vi "nanocal -- nuclear schottky fit -- 2x2 -- V9.vi"() -> ()   [LabVIEW 2021] (continued)
\"τC\" -> 0.000000000000   ,  \"κ0\" -> 0.000000000000   ,  \"mm1\" -> 0.000000000000   ,  \"mm2\" -> 0.000000000000   ,  \"mm3\" -> 0.000000000000   ,  \"T\" -> 3.070000000000   ,  \"B\" -> 4.000000000000   ,  \"θ\" -> 0.000000000000   ,  \"Reoff\" -> 0.000000000000   ,  \"Imoff\" -> 0.000000000000   ,  \"στ1\" -> 0.000000000000   ,  \"στS\" -> 0.000000000000   ,  \"στN\" -> 0.000000000000    |>   , \r\"IDS0473_220531_RAW_cal__ref_\" ->   <|    \"ζ\" -> 0.022738475228   ,  \"τ1\" -> 0.084920254079   ,  \"τS\" -> 0.005823220552   ,  \"τN\" -> 0.000435197334   ,  \"τC\" -> 0.002070516453   ,  \"κ0\" -> 0.000000054886   ,  \"mm1\" -> 0.000034304647   ,  \"mm2\" -> 0.007945964933   ,  \"mm3\" -> 0.085411225719   ,  \"T\" -> 5.700000000000   ,  \"B\" -> 4.000000000000   ,  \"θ\" -> 0.000000000000   ,  \"Reoff\" -> -102040.816326530650   ,  \"Imoff\" -> 0.000000000000   ,  \"στ1\" -> 0.009006871180   ,  \"στS\" -> 0.000077078263   ,  \"στN\" -> 0.000007381756    |>   , \r\"IDS0473_220531_RAW_cal__sam_\" ->   <|    \"ζ\" -> 0.000000000000   ,  \"τ1\" -> 0.000000000000   ,  \"τS\" -> 0.000000000000   ,  \"τN\" -> 0.000000000000   ,  \"τC\" -> 0.000000000000   ,  \"κ0\" -> 0.000000000000   ,  \"mm1\" -> 0.000000000000   ,  \"mm2\" -> 0.000000000000   ,  \"mm3\" -> 0.000000000000   ,  \"T\" -> 5.700000000000   ,  \"B\" -> 4.000000000000   ,  \"θ\" -> 0.000000000000   ,  \"Reoff\" -> 0.000000000000   ,  \"Imoff\" -> 0.000000000000   ,  \"στ1\" -> 0.000000000000   ,  \"στS\" -> 0.000000000000   ,  \"στN\" -> 0.000000000000    |>   , \r\"IDS0477_220601_RAW_cal__ref_\" ->   <|    \"ζ\" -> 0.239805642697   ,  \"τ1\" -> 0.033790664831   ,  \"τS\" -> 0.059024379220   ,  \"τN\" -> 0.060427064379   ,  \"τC\" -> 0.000896937980   ,  \"κ0\" -> 0.000000000920   ,  \"mm1\" -> 0.000171776345   ,  \"mm2\" -> 0.014890032084   ,  \"mm3\" -> 0.167722368184   ,  \"T\" -> 0.200000000000   ,  \"B\" -> 10.000000000000   ,  \"θ\" -> 45.000000000000   ,  \"Reoff\" -> -36122448.979591839000   ,  \"Imoff\" -> 0.000000000000   ,  \"στ1\" -> 0.011907202865   ,  \"στS\" -> 0.006392080806   ,  \"στN\" -> 0.010956766376    |>   , \r\"IDS0477_220601_RAW_cal__sam_\" ->   <|    \"ζ\" -> 0.000000000000   ,  \"τ1\" -> 0.000000000000   ,  \"τS\" -> 0.000000000000   ,  \"τN\" -> 0.000000000000   ,  \"τC\" -> 0.000000000000   ,  \"κ0\" -> 0.000000000000   ,  \"mm1\" -> 0.000000000000   ,  \"mm2\" -> 0.000000000000   ,  \"mm3\" -> 0.000000000000   ,  \"T\" -> 0.200000000000   ,  \"B\" -> 10.000000000000   ,  \"θ\" -> 45.000000000000   ,  \"Reoff\" -> 0.000000000000   ,  \"Imoff\" -> 0.000000000000   ,  \"στ1\" -> 0.000000000000   ,  \"στS\" -> 0.000000000000   ,  \"στN\" -> 0.000000000000    |>   , \r\"IDS0478_220601_RAW_cal__ref_\" ->   <|    \"ζ\" -> 0.152803180528   ,  \"τ1\" -> 0.028187868792   ,  \"τS\" -> 0.047098340694   ,  \"τN\" -> 0.025207837056   ,  \"τC\" -> 0.000982024605   ,  \"κ0\" -> 0.000000001260   ,  \"mm1\" -> 0.000128146365   ,  \"mm2\" -> 0.016152622122   ,  \"mm3\" -> 0.096243916593   ,  \"T\" -> 0.250000000000   ,  \"B\" -> 10.000000000000   ,  \"θ\" -> 45.000000000000   ,  \"Reoff\" -> -18163265.306122452000   ,  \"Imoff\" -> 0.000000000000   ,  \"στ1\" -> 0.005041045857   ,  \"στS\" -> 0.001567344139   ,  \"στN\" -> 0.002277988599    |>   , \r\"IDS0478_220601_RAW_cal__sam_\" ->   <|    \"ζ\" -> 0.000000000000   ,  \"τ1\" -> 0.000000000000   ,  \"τS\" -> 0.000000000000   ,  \"τN\" -> 0.000000000000   ,  \"τC\" -> 0.000000000000   ,  \"κ0\" -> 0.000000000000   ,  \"mm1\" -> 0.000000000000   ,  \"mm2\" -> 0.000000000000   ,  \"mm3\" -> 0.000000000000   ,  \"T\" -> 0.250000000000   ,  \"B\" -> 10.000000000000   ,  \"θ\" -> 45.000000000000   ,  \"Reoff\" -> 0.000000000000   ,  \"Imoff\" -> 0.000000000000   ,  \"στ1\" -> 0.000000000000   ,  \"στS\" -> 0.000000000000   ,  \"στN\" -> 0.000000000000    |>   , \r\"IDS0479_220601_RAW_cal__ref_\" ->   <|    \"ζ\" -> 0.111193066205   ,  \"τ1\" -> 0.024122553376   ,  \"τS\" -> 0.042118651402   ,  \"τN\" -> 0.013651970206   ,  \"τC\" -> 0.001072327817   ,  \"κ0\" -> 0.000000001570   ,  \"mm1\" -> 0.000105128315   ,  \"mm2\" -> 0.016280391263   ,  \"mm3\" -> 0.070781289644   ,  \"T\" -> 0.300000000000   ,  \"B\" -> 10.000000000000   ,  \"θ\" -> 45.000000000000   ,  \"Reoff\" -> -10816326.530612245200   ,  \"Imoff\" -> 0.000000000000   ,  \"στ1\" -> 0.003531051170   ,  \"στS\" -> 0.000678989919   ,  \"στN\" -> 0.000877996668    |>   , \r\"IDS0479_220601_RAW_cal__sam_\" ->   <|    \"ζ\" -> 0.000000000000   ,  \"τ1\" -> 0.000000000000   ,  \"τS\" -> 0.000000000000   ,  \"τN\" -> 0.000000000000   ,  \"τC\" -> 0.000000000000   ,  \"κ0\" -> 0.000000000000   ,  \"mm1\" -> 0.000000000000   ,  \"mm2\" -> 0.000000000000   ,  \"mm3\" -> 0.000000000000   ,  \"T\" -> 0.300000000000   ,  \"B\" -> 10.000000000000   ,  \"θ\" -> 45.000000000000   ,  \"Reoff\" -> 0.000000000000   ,  \"Imoff\" -> 0.000000000000   ,  \"στ1\" -> 0.000000000000   ,  \"στS\" -> 0.000000000000   ,  \"στN\" -> 0.000000000000    |>   , \r\"IDS0480_220601_RAW_cal__ref_\" ->   <|    \"ζ\" -> 0.079231560459   ,  \"τ1\" -> 0.017107381840   ,  \"τS\" -> 0.036891145607   ,  \"τN\" -> 0.007202328301   ,  \"τC\" -> 0.001264563258   ,  \"κ0\" -> 0.000000002000   ,  \"mm1\" -> 0.000090175019   ,  \"mm2\" -> 0.013352548983   ,  \"mm3\" -> 0.052516289748   ,  \"T\" -> 0.360000000000   ,  \"B\" -> 10.000000000000   ,  \"θ\" -> 45.000000000000   ,  \"Reoff\" -> -6326530.612244904040   ,  \"Imoff\" -> 0.000000000000   ,  \"στ1\" -> 0.001933309697   ,  \"στS\" -> 0.000284795622   ,  \"στN\" -> 0.000344056722    |>   , \r\"IDS0480_220601_RAW_cal__sam_\" ->   <|    \"ζ\" -> 0.000000000000   ,  \"τ1\" -> 0.000000000000   ,  \"τS\" -> 0.000000000000   ,  \"τN\" -> 0.000000000000   ,  \"τC\" -> 0.000000000000   ,  \"κ0\" -> 0.000000000000   ,  \"mm1\" -> 0.000000000000   ,  \"mm2\" -> 0.000000000000   ,  \"mm3\" -> 0.000000000000   ,  \"T\" -> 0.360000000000   ,  \"B\" -> 10.000000000000   ,  \"θ\" -> 45.000000000000   ,  \"Reoff\" -> 0.000000000000   ,  \"Imoff\" -> 0.000000000000   ,  \"στ1\" -> 0.000000000000   ,  \"στS\" -> 0.000000000000   ,  \"στN\" -> 0.000000000000    |>   , \r\"IDS0481_220601_RAW_cal__ref_\" ->   <|    \"ζ\" -> 0.059346185114   ,  \"τ1\" -> 0.015969775027   ,  \"τS\" -> 0.034144098652   ,  \"τN\" -> 0.004294468384   ,  \"τC\" -> 0.001604549811   ,  \"κ0\" -> 0.000000002410   ,  \"mm1\" -> 0.000086265768   ,  \"mm2\" -> 0.013446939913   ,  \"mm3\" -> 0.044760868507   ,  \"T\" -> 0.420000000000   ,  \"B\" -> 10.000000000000   ,  \"θ\" -> 45.000000000000   ,  \"Reoff\" -> -3061224.489795923230   ,  \"Imoff\" -> 0.000000000000   ,  \"στ1\" -> 0.000907344416   ,  \"στS\" -> 0.000176030005   ,  \"στN\" -> 0.000148751487    |>   , \r\"IDS0481_220601_RAW_cal__sam_\" ->   <|    \"ζ\" -> 0.000000000000   ,  \"τ1\" -> 0.000000000000   ,  \"τS\" -> 0.000000000000   ,  \"τN\" -> 0.000000000000   ,  \"τC\" -> 0.000000000000   ,  \"κ0\" -> 0.000000000000   ,  \"mm1\" -> 0.000000000000   ,  \"mm2\" -> 0.000000000000   ,  \"mm3\" -> 0.000000000000   ,  \"T\" -> 0.420000000000   ,  \"B\" -> 10.000000000000   ,  \"θ\" -> 45.000000000000   ,  \"Reoff\" -> 0.000000000000   ,  \"Imoff\" -> 0.000000000000   ,  \"στ1\" -> 0.000000000000   ,  \"στS\" -> 0.000000000000   ,  \"στN\" -> 0.000000000000    |>   , \r\"IDS0482_220601_RAW_cal__ref_\" ->   <|    \"ζ\" -> 0.043142553496   ,  \"τ1\" -> 0.014499389185   ,  \"τS\" -> 0.030371945733   ,  \"τN\" -> 0.002402650316   ,  \"τC\" -> 0.001877907190   ,  \"κ0\" -> 0.000000003100   ,  \"mm1\" -> 0.000073480289   ,  \"mm2\" -> 0.012924539137   ,  \"mm3\" -> 0.037567852762   ,  \"T\" -> 0.520000000000   ,  \"B\" -> 10.000000000000   ,  \"θ\" -> 45.000000000000   ,  \"Reoff\" -> -1836734.693877555430   ,  \"Imoff\" -> 0.000000000000   ,  \"στ1\" -> 0.000488095502   ,  \"στS\" -> 0.000097405917   ,  \"στN\" -> 0.000051506778    |>   , \r\"IDS0482_220601_RAW_cal__sam_\" ->   <|    \"ζ\" -> 0.000000000000   ,  \"τ1\" -> 0.000000000000   ,  \"τS\" -> 0.000000000000   ,  \"τN\" -> 0.000000000000   ,  \"τC\" -> 0.000000000000   ,  \"κ0\" -> 0.000000000000   ,  \"mm1\" -> 0.000000000000   ,  \"mm2\" -> 0.000000000000   ,  \"mm3\" -> 0.000000000000   ,  \"T\" -> 0.520000000000   ,  \"B\" -> 10.000000000000   ,  \"θ\" -> 45.000000000000   ,  \"Reoff\" -> 0.000000000000   ,  \"Imoff\" -> 0.000000000000   ,  \"στ1\" -> 0.000000000000   ,  \"στS\" -> 0.000000000000   ,  \"στN\" -> 0.000000000000    |>   , \r\"IDS0483_220601_RAW_cal__ref_\" ->   <|    \"ζ\" -> 0.037957534412   ,  \"τ1\" -> 0.013025982486   ,  \"τS\" -> 0.027861955043   ,  \"τN\" -> 0.001482537125   ,  \"τC\" -> 0.001562153050   ,  \"κ0\" -> 0.000000003750   ,  \"mm1\" -> 0.000054295490   ,  \"mm2\" -> 0.012021211304   ,  \"mm3\" -> 0.032970965481   ,  \"T\" -> 0.620000000000   ,  \"B\" -> 10.000000000000   ,  \"θ\" -> 45.000000000000   ,  \"Reoff\" -> -2489795.918367348610   ,  \"Imoff\" -> 0.000000000000   ,  \"στ1\" -> 0.000872811735   ,  \"στS\" -> 0.000114206450   ,  \"στN\" -> 0.000055407234    |>   , \r\"IDS0483_220601_RAW_cal__sam_\" ->   <|    \"ζ\" -> 0.000000000000   ,  \"τ1\" -> 0.000000000000   ,  \"τS\" -> 0.000000000000   ,  \"τN\" -> 0.000000000000   ,  \"τC\" -> 0.000000000000   ,  \"κ0\" -> 0.000000000000   ,  \"mm1\" -> 0.000000000000   ,  \"mm2\" -> 0.000000000000   ,  \"mm3\" -> 0.000000000000   ,  \"T\" -> 0.620000000000   ,  \"B\" -> 10.000000000000   ,  \"θ\" -> 45.000000000000   ,  \"Reoff\" -> 0.000000000000   ,  \"Imoff\" -> 0.000000000000   ,  \"στ1\" -> 0.000000000000   ,  \"στS\" -> 0.000000000000   ,  \"στN\" -> 0.000000000000    |>   , \r\"IDS0484_220601_RAW_cal__ref_\" ->   <|    \"ζ\" -> 0.026779879048   ,  \"τ1\" -> 0.012724854717   ,  \"τS\" -> 0.023406495826   ,  \"τN\" -> 0.000845574693   ,  \"τC\" -> 0.002190018434   ,  \"κ0\" -> 0.000000005114   ,  \"mm1\" -> 0.000052452848   ,  \"mm2\" -> 0.011990951083   ,  \"mm3\" -> 0.027773007254   ,  \"T\" -> 0.820000000000   ,  \"B\" -> 10.000000000000   ,  \"θ\" -> 45.000000000000   ,  \"Reoff\" -> -1020408.163265310230   ,  \"Imoff\" -> 0.000000000000   ,  \"στ1\" -> 0.000585844678   ,  \"στS\" -> 0.000123901377   ,  \"στN\" -> 0.000022627070    |>   , \r\"IDS0484_220601_RAW_cal__sam_\" ->   <|    \"ζ\" -> 0.000000000000   ,  \"τ1\" -> 0.000000000000   ,  \"τS\" -> 0.000000000000   ,  \"τN\" -> 0.000000000000   ,  \"τC\" -> 0.000000000000   ,  \"κ0\" -> 0.000000000000   ,  \"mm1\" -> 0.000000000000   ,  \"mm2\" -> 0.000000000000   ,  \"mm3\" -> 0.000000000000   ,  \"T\" -> 0.820000000000   ,  \"B\" -> 10.000000000000   ,  \"θ\" -> 45.000000000000   ,  \"Reoff\" -> 0.000000000000   ,  \"Imoff\" -> 0.000000000000   ,  \"στ1\" -> 0.000000000000   ,  \"στS\" -> 0.000000000000   ,  \"στN\" -> 0.000000000000    |>   , \r\"IDS0485_220601_RAW_cal__ref_\" ->   <|    \"ζ\" -> 0.326622885443   ,  \"τ1\" -> 0.044212332753   ,  \"τS\" -> 0.078119393187   ,  \"τN\" -> 0.109436103453   ,  \"τC\" -> 0.000856629079   ,  \"κ0\" -> 0.000000000725   ,  \"mm1\" -> 0.000209590105   ,  \"mm2\" -> 0.016643396508   ,  \"mm3\" -> 0.277031389353   ,  \"T\" -> 0.170000000000   ,  \"B\" -> 10.000000000000   ,  \"θ\" -> 45.000000000000   ,  \"Reoff\" -> -62040816.326530613000   ,  \"Imoff\" -> 0.000000000000   ,  \"στ1\" -> 0.024054965225   ,  \"στS\" -> 0.017110063636   ,  \"στN\" -> 0.032486922745    |>   , \r\"IDS0485_220601_RAW_cal__sam_\" ->   <|    \"ζ\" -> 0.000000000000   ,  \"τ1\" -> 0.000000000000   ,  \"τS\" -> 0.000000000000   ,  \"τN\" -> 0.000000000000   ,  \"τC\" -> 0.000000000000   ,  \"κ0\" -> 0.000000000000   ,  \"mm1\" -> 0.000000000000   ,  \"mm2\" -> 0.000000000000   ,  \"mm3\" -> 0.000000000000   ,  \"T\" -> 0.170000000000   ,  \"B\" -> 10.000000000000   ,  \"θ\" -> 45.000000000000   ,  \"Reoff\" -> 0.000000000000   ,  \"Imoff\" -> 0.000000000000   ,  \"στ1\" -> 0.000000000000   ,  \"στS\" -> 0.000000000000   ,  \"στN\" -> 0.000000000000    |>   , \r\"IDS0486_220602_RAW_cal__ref_\" ->   <|    \"ζ\" -> 0.649293881953   ,  \"τ1\" -> 0.043625300429   ,  \"τS\" -> 0.134917071733   ,  \"τN\" -> 0.437947607875   ,  \"τC\" -> 0.000801229494   ,  \"κ0\" -> 0.000000000457   ,  \"mm1\" -> 0.000314723238   ,  \"mm2\" -> 0.009937880875   ,  \"mm3\" -> 0.978996137075   ,  \"T\" -> 0.120000000000   ,  \"B\" -> 10.000000000000   ,  \"θ\" -> 45.000000000000   ,  \"Reoff\" -> -171836734.693877578000   ,  \"Imoff\" -> 0.000000000000   ,  \"στ1\" -> 0.033288763136   ,  \"στS\" -> 0.058140913362   ,  \"στN\" -> 0.147341239880    |>   , \r\"IDS0486_220602_RAW_cal__sam_\" ->   <|    \"ζ\" -> 0.000000000000   ,  \"τ1\" -> 0.000000000000   ,  \"τS\" -> 0.000000000000   ,  \"τN\" -> 0.000000000000   ,  \"τC\" -> 0.000000000000   ,  \"κ0\" -> 0.000000000000   ,  \"mm1\" -> 0.000000000000   ,  \"mm2\" -> 0.000000000000   ,  \"mm3\" -> 0.000000000000   ,  \"T\" -> 0.120000000000   ,  \"B\" -> 10.000000000000   ,  \"θ\" -> 45.000000000000   ,  \"Reoff\" -> 0.000000000000   ,  \"Imoff\" -> 0.000000000000   ,  \"στ1\" -> 0.000000000000   ,  \"στS\" -> 0.000000000000   ,  \"στN\" -> 0.000000000000    |>   , \r\"IDS0487_220602_RAW_cal__ref_\" ->   <|    \"ζ\" -> 0.408039702366   ,  \"τ1\" -> 0.042905840355   ,  \"τS\" -> 0.097971452964   ,  \"τN\" -> 0.156381067039   ,  \"τC\" -> 0.000853577753   ,  \"κ0\" -> 0.000000000645   ,  \"mm1\" -> 0.000246266382   ,  \"mm2\" -> 0.015391335627   ,  \"mm3\" -> 0.386260262660   ,  \"T\" -> 0.150000000000   ,  \"B\" -> 10.000000000000   ,  \"θ\" -> 45.000000000000   ,  \"Reoff\" -> -71428571.428571432800   ,  \"Imoff\" -> 0.000000000000   ,  \"στ1\" -> 0.036951115760   ,  \"στS\" -> 0.039139419252   ,  \"στN\" -> 0.072533278240    |>   , \r\"IDS0487_220602_RAW_cal__sam_\" ->   <|    \"ζ\" -> 0.000000000000   ,  \"τ1\" -> 0.000000000000   ,  \"τS\" -> 0.000000000000   ,  \"τN\" -> 0.000000000000   ,  \"τC\" -> 0.000000000000   ,  \"κ0\" -> 0.000000000000   ,  \"mm1\" -> 0.000000000000   ,  \"mm2\" -> 0.000000000000   ,  \"mm3\" -> 0.000000000000   ,  \"T\" -> 0.150000000000   ,  \"B\" -> 10.000000000000   ,  \"θ\" -> 45.000000000000   ,  \"Reoff\" -> 0.000000000000   ,  \"Imoff\" -> 0.000000000000   ,  \"στ1\" -> 0.000000000000   ,  \"στS\" -> 0.000000000000   ,  \"στN\" -> 0.000000000000    |>   , \r\"IDS0488_220602_RAW_cal__ref_\" ->   <|    \"ζ\" -> 0.022173506919   ,  \"τ1\" -> 0.011885040231   ,  \"τS\" -> 0.019213986471   ,  \"τN\" -> 0.000342476634   ,  \"τC\" -> 0.002250605678   ,  \"κ0\" -> 0.000000007250   ,  \"mm1\" -> 0.000043889604   ,  \"mm2\" -> 0.011496376729   ,  \"mm3\" -> 0.022585478052   ,  \"T\" -> 1.120000000000   ,  \"B\" -> 10.000000000000   ,  \"θ\" -> 45.000000000000   ,  \"Reoff\" -> -775510.204081632196   ,  \"Imoff\" -> 0.000000000000   ,  \"στ1\" -> 0.000592033773   ,  \"στS\" -> 0.000127596201   ,  \"στN\" -> 0.000006161863    |>   , \r\"IDS0488_220602_RAW_cal__sam_\" ->   <|    \"ζ\" -> 0.000000000000   ,  \"τ1\" -> 0.000000000000   ,  \"τS\" -> 0.000000000000   ,  \"τN\" -> 0.000000000000   ,  \"τC\" -> 0.000000000000   ,  \"κ0\" -> 0.000000000000   ,  \"mm1\" -> 0.000000000000   ,  \"mm2\" -> 0.000000000000   ,  \"mm3\" -> 0.000000000000   ,  \"T\" -> 1.120000000000   ,  \"B\" -> 10.000000000000   ,  \"θ\" -> 45.000000000000   ,  \"Reoff\" -> 0.000000000000   ,  \"Imoff\" -> 0.000000000000   ,  \"στ1\" -> 0.000000000000   ,  \"στS\" -> 0.000000000000   ,  \"στN\" -> 0.000000000000    |>   , \r\"IDS0489_220602_RAW_cal__ref_\" ->   <|    \"ζ\" -> 0.017612684006   ,  \"τ1\" -> 0.012096462763   ,  \"τS\" -> 0.012962092030   ,  \"τN\" -> 0.000222284463   ,  \"τC\" -> 0.003088642356   ,  \"κ0\" -> 0.000000012650   ,  \"mm1\" -> 0.000043430503   ,  \"mm2\" -> 0.011540887541   ,  \"mm3\" -> 0.017017375825   ,  \"T\" -> 1.900000000000   ,  \"B\" -> 10.000000000000   ,  \"θ\" -> 45.000000000000   ,  \"Reoff\" -> -285714.285714283585   ,  \"Imoff\" -> 0.000000000000   ,  \"στ1\" -> 0.000551045150   ,  \"στS\" -> 0.000068203719   ,  \"στN\" -> 0.000001106043    |>   , \r\"IDS0489_220602_RAW_cal__sam_\" ->   <|    \"ζ\" -> 0.000000000000   ,  \"τ1\" -> 0.000000000000   ,  \"τS\" -> 0.000000000000   ,  \"τN\" -> 0.000000000000   ,  \"τC\" -> 0.000000000000   ,  \"κ0\" -> 0.000000000000   ,  \"mm1\" -> 0.000000000000   ,  \"mm2\" -> 0.000000000000   ,  \"mm3\" -> 0.000000000000   ,  \"T\" -> 1.900000000000   ,  \"B\" -> 10.000000000000   ,  \"θ\" -> 45.000000000000   ,  \"Reoff\" -> 0.000000000000   ,  \"Imoff\" -> 0.000000000000   ,  \"στ1\" -> 0.000000000000   ,  \"στS\" -> 0.000000000000   ,  \"στN\" -> 0.000000000000    |>   , \r\"IDS0490_220602_RAW_cal__ref_\" ->   <|    \"ζ\" -> 0.017543790991   ,  \"τ1\" -> 0.012306369906   ,  \"τS\" -> 0.009201126322   ,  \"τN\" -> 0.000228437361   ,  \"τC\" -> 0.002737880162   ,  \"κ0\" -> 0.000000022450   ,  \"mm1\" -> 0.000036634285   ,  \"mm2\" -> 0.010610708634   ,  \"mm3\" -> 0.013991901127   ,  \"T\" -> 3.100000000000   ,  \"B\" -> 10.000000000000   ,  \"θ\" -> 45.000000000000   ,  \"Reoff\" -> -204081.632653061300   ,  \"Imoff\" -> 0.000000000000   ,  \"στ1\" -> 0.002672802022   ,  \"στS\" -> 0.000083863573   ,  \"στN\" -> 0.000016880987    |>   , \r\"IDS0490_220602_RAW_cal__sam_\" ->   <|    \"ζ\" -> 0.000000000000   ,  \"τ1\" -> 0.000000000000   ,  \"τS\" -> 0.000000000000   ,  \"τN\" -> 0.000000000000   ,  \"τC\" -> 0.000000000000   ,  \"κ0\" -> 0.000000000000   ,  \"mm1\" -> 0.000000000000   ,  \"mm2\" -> 0.000000000000   ,  \"mm3\" -> 0.000000000000   ,  \"T\" -> 3.100000000000   ,  \"B\" -> 10.000000000000   ,  \"θ\" -> 45.000000000000   ,  \"Reoff\" -> 0.000000000000   ,  \"Imoff\" -> 0.000000000000   ,  \"στ1\" -> 0.000000000000   ,  \"στS\" -> 0.000000000000   ,  \"στN\" -> 0.000000000000    |>   , \r"
  in  "string IN":string="  \"IDS0158_210310_RAW_cal__ref_\" ->   <|    \"ζ\" -> 0.338724462580   ,  \"τ1\" -> 0.031757745266   ,  \"τS\" -> 0.247286819047   ,  \"τN\" -> 0.322740818116   ,  \"τC\" -> 0.001034291318   ,  \"κ0\" -> 0.000000000505   ,  \"mm1\" -> 0.000261080239   ,  \"mm2\" -> 0.013473055910   ,  \"mm3\" -> 0.782167842652   ,  \"T\" -> 0.120000000000   ,  \"B\" -> 12.000000000000   ,  \"θ\" -> 0.000000000000   ,  \"Reoff\" -> -114641566.265060246000   ,  \"Imoff\" -> 0.000000000000   ,  \"στ1\" -> 0.033488050442   ,  \"στS\" -> 0.029896570326   ,  \"στN\" -> 0.000000000000    |>   , \n\"IDS0158_210310_RAW_cal__sam_\" ->   <|    \"ζ\" -> 0.286336668596   ,  \"τ1\" -> 0.037477267671   ,  \"τS\" -> 0.354459287884   ,  \"τN\" -> 0.444916383639   ,  \"τC\" -> 0.001225600579   ,  \"κ0\" -> 0.000000000596   ,  \"mm1\" -> 0.000272242393   ,  \"mm2\" -> 0.016302418461   ,  \"mm3\" -> 1.050394445660   ,  \"T\" -> 0.120000000000   ,  \"B\" -> 12.000000000000   ,  \"θ\" -> 0.000000000000   ,  \"Reoff\" -> 0.000000000000   ,  \"Imoff\" -> 0.000000000000   ,  \"στ1\" -> 0.000000000000   ,  \"στS\" -> 0.000000000000   ,  \"στN\" -> 0.000000000000    |>   , \n\"IDS0159_210310_RAW_cal__ref_\" ->   <|    \"ζ\" -> 0.271267920492   ,  \"τ1\" -> 0.029985631647   ,  \"τS\" -> 0.193691005295   ,  \"τN\" -> 0.182171075098   ,  \"τC\" -> 0.001008816819   ,  \"κ0\" -> 0.000000000648   ,  \"mm1\" -> 0.000214568285   ,  \"mm2\" -> 0.015007137955   ,  \"mm3\" -> 0.493594147559   ,  \"T\" -> 0.150000000000   ,  \"B\" -> 12.000000000000   ,  \"θ\" -> 0.000000000000   ,  \"Reoff\" -> -68518072.289156615700   ,  \"Imoff\" -> 0.000000000000   ,  \"στ1\" -> 0.012908928279   ,  \"στS\" -> 0.012278249433   ,  \"στN\" -> 0.000000000000    |>   , \n\"IDS0159_210310_RAW_cal__sam_\" ->   <|    \"ζ\" -> 0.219100303741   ,  \"τ1\" -> 0.028643012604   ,  \"τS\" -> 0.279362928811   ,  \"τN\" -> 0.246156444058   ,  \"τC\" -> 0.001272401549   ,  \"κ0\" -> 0.000000000760   ,  \"mm1\" -> 0.000227975653   ,  \"mm2\" -> 0.014929571562   ,  \"mm3\" -> 0.655418694024   ,  \"T\" -> 0.150000000000   ,  \"B\" -> 12.000000000000   ,  \"θ\" -> 0.000000000000   ,  \"Reoff\" -> 0.000000000000   ,  \"Imoff\" -> 0.000000000000   ,  \"στ1\" -> 0.000000000000   ,  \"στS\" -> 0.000000000000   ,  \"στN\" -> 0.000000000000    |>   , \n\"IDS0160_210310_RAW_cal__ref_\" ->   <|    \"ζ\" -> 0.207139977904   ,  \"τ1\" -> 0.027467343957   ,  \"τS\" -> 0.117438673826   ,  \"τN\" -> 0.102057074143   ,  \"τC\" -> 0.000949663971   ,  \"κ0\" -> 0.000000000917   ,  \"mm1\" -> 0.000162053218   ,  \"mm2\" -> 0.014024936030   ,  \"mm3\" -> 0.279192111033   ,  \"T\" -> 0.180000000000   ,  \"B\" -> 12.000000000000   ,  \"θ\" -> 0.000000000000   ,  \"Reoff\" -> -40668674.698795177000   ,  \"Imoff\" -> 0.000000000000   ,  \"στ1\" -> 0.009618369087   ,  \"στS\" -> 0.007137384425   ,  \"στN\" -> 0.000000000000    |>   , \n\"IDS0160_210310_RAW_cal__sam_\" ->   <|    \"ζ\" -> 0.170488637524   ,  \"τ1\" -> 0.029234231120   ,  \"τS\" -> 0.149095458227   ,  \"τN\" -> 0.151792620275   ,  \"τC\" -> 0.001113424175   ,  \"κ0\" -> 0.000000001042   ,  \"mm1\" -> 0.000161291869   ,  \"mm2\" -> 0.013922632736   ,  \"mm3\" -> 0.368449807743   ,  \"T\" -> 0.180000000000   ,  \"B\" -> 12.000000000000   ,  \"θ\" -> 0.000000000000   ,  \"Reoff\" -> 0.000000000000   ,  \"Imoff\" -> 0.000000000000   ,  \"στ1\" -> 0.000000000000   ,  \"στS\" -> 0.000000000000   ,  \"στN\" -> 0.000000000000    |>   , \n\"IDS0161_210310_RAW_cal__ref_\" ->   <|    \"ζ\" -> 0.165651103495   ,  \"τ1\" -> 0.025219369633   ,  \"τS\" -> 0.095243887499   ,  \"τN\" -> 0.068405844588   ,  \"τC\" -> 0.001096621932   ,  \"κ0\" -> 0.000000001058   ,  \"mm1\" -> 0.000154524257   ,  \"mm2\" -> 0.013909362731   ,  \"mm3\" -> 0.203010595371   ,  \"T\" -> 0.200000000000   ,  \"B\" -> 12.000000000000   ,  \"θ\" -> 0.000000000000   ,  \"Reoff\" -> -26138554.216867461800   ,  \"Imoff\" -> 0.000000000000   ,  \"στ1\" -> 0.007587881902   ,  \"στS\" -> 0.004844828321   ,  \"στN\" -> 0.000000000000    |>   , \n\"IDS0161_210310_RAW_cal__sam_\" ->   <|    \"ζ\" -> 0.130531197151   ,  \"τ1\" -> 0.025704482770   ,  \"τS\" -> 0.129606657196   ,  \"τN\" -> 0.091602369165   ,  \"τC\" -> 0.001441379995   ,  \"κ0\" -> 0.000000001211   ,  \"mm1\" -> 0.000164978070   ,  \"mm2\" -> 0.014468182937   ,  \"mm3\" -> 0.262596407151   ,  \"T\" -> 0.200000000000   ,  \"B\" -> 12.000000000000   ,  \"θ\" -> 0.000000000000   ,  \"Reoff\" -> 0.000000000000   ,  \"Imoff\" -> 0.000000000000   ,  \"στ1\" -> 0.000000000000   ,  \"στS\" -> 0.000000000000   ,  \"στN\" -> 0.000000000000    |>   , \n\"IDS0162_210310_RAW_cal__ref_\" ->   <|    \"ζ\" -> 0.096222034275   ,  \"τ1\" -> 0.023686784650   ,  \"τS\" -> 0.070336744639   ,  \"τN\" -> 0.023939989572   ,  \"τC\" -> 0.001388596335   ,  \"κ0\" -> 0.000000001367   ,  \"mm1\" -> 0.000119909077   ,  \"mm2\" -> 0.016622969082   ,  \"mm3\" -> 0.111680736187   ,  \"T\" -> 0.250000000000   ,  \"B\" -> 12.000000000000   ,  \"θ\" -> 0.000000000000   ,  \"Reoff\" -> -11003012.048192769300   ,  \"Imoff\" -> 0.000000000000   ,  \"στ1\" -> 0.008753356754   ,  \"στS\" -> 0.002669913437   ,  \"στN\" -> 0.000000000000    |>   , \n\"IDS0162_210310_RAW_cal__sam_\" ->   <|    \"ζ\" -> 0.078258046754   ,  \"τ1\" -> 0.028009840731   ,  \"τS\" -> 0.092122038762   ,  \"τN\" -> 0.030129595899   ,  \"τC\" -> 0.001641062244   ,  \"κ0\" -> 0.000000001543   ,  \"mm1\" -> 0.000117303440   ,  \"mm2\" -> 0.019983073008   ,  \"mm3\" -> 0.141369335330   ,  \"T\" -> 0.250000000000   ,  \"B\" -> 12.000000000000   ,  \"θ\" -> 0.000000000000   ,  \"Reoff\" -> 0.000000000000   ,  \"Imoff\" -> 0.000000000000   ,  \"στ1\" -> 0.000000000000   ,  \"στS\" -> 0.000000000000   ,  \"στN\" -> 0.000000000000    |>   , \n\"IDS0163_210310_RAW_cal__ref_\" ->   <|    \"ζ\" -> 0.066672200447   ,  \"τ1\" -> 0.021639337174   ,  \"τS\" -> 0.054330230678   ,  \"τN\" -> 0.012190158529   ,  \"τC\" -> 0.001673698086   ,  \"κ0\" -> 0.000000001744   ,  \"mm1\" -> 0.000101848885   ,  \"mm2\" -> 0.016608176692   ,  \"mm3\" -> 0.077558459612   ,  \"T\" -> 0.300000000000   ,  \"B\" -> 12.000000000000   ,  \"θ\" -> 0.000000000000   ,  \"Reoff\" -> -6192771.084337353710   ,  \"Imoff\" -> 0.000000000000   ,  \"στ1\" -> 0.010795838687   ,  \"στS\" -> 0.002003612837   ,  \"στN\" -> 0.000000000000    |>   , \n\"IDS0163_210310_RAW_cal__sam_\" ->   <|    \"ζ\" -> 0.054088186012   ,  \"τ1\" -> 0.023838802615   ,  \"τS\" -> 0.069079396629   ,  \"τN\" -> 0.016435267456   ,  \"τC\" -> 0.002025071743   ,  \"κ0\" -> 0.000000001955   ,  \"mm1\" -> 0.000101234646   ,  \"mm2\" -> 0.018244822177   ,  \"mm3\" -> 0.097657814678   ,  \"T\" -> 0.300000000000   ,  \"B\" -> 12.000000000000   ,  \"θ\" -> 0.000000000000   ,  \"Reoff\" -> 0.000000000000   ,  \"Imoff\" -> 0.000000000000   ,  \"στ1\" -> 0.000000000000   ,  \"στS\" -> 0.000000000000   ,  \"στN\" -> 0.000000000000    |>   , \n\"IDS0164_210310_RAW_cal__ref_\" ->   <|    \"ζ\" -> 0.047185670549   ,  \"τ1\" -> 0.020999787986   ,  \"τS\" -> 0.044123234525   ,  \"τN\" -> 0.006414229914   ,  \"τC\" -> 0.002330922094   ,  \"κ0\" -> 0.000000002161   ,  \"mm1\" -> 0.000100189786   ,  \"mm2\" -> 0.017276594586   ,  \"mm3\" -> 0.058876034294   ,  \"T\" -> 0.360000000000   ,  \"B\" -> 12.000000000000   ,  \"θ\" -> 0.000000000000   ,  \"Reoff\" -> -3126506.024096369740   ,  \"Imoff\" -> 0.000000000000   ,  \"στ1\" -> 0.014319461595   ,  \"στS\" -> 0.001588428387   ,  \"στN\" -> 0.000000000000    |>   , \n\"IDS0164_210310_RAW_cal__sam_\" ->   <|    \"ζ\" -> 0.039314966212   ,  \"τ1\" -> 0.020712803909   ,  \"τS\" -> 0.055413767550   ,  \"τN\" -> 0.008474403424   ,  \"τC\" -> 0.002674063387   ,  \"κ0\" -> 0.000000002415   ,  \"mm1\" -> 0.000096818147   ,  \"mm2\" -> 0.017190811405   ,  \"mm3\" -> 0.072499170001   ,  \"T\" -> 0.360000000000   ,  \"B\" -> 12.000000000000   ,  \"θ\" -> 0.000000000000   ,  \"Reoff\" -> 0.000000000000   ,  \"Imoff\" -> 0.000000000000   ,  \"στ1\" -> 0.000000000000   ,  \"στS\" -> 0.000000000000   ,  \"στN\" -> 0.000000000000    |>   , \n\"IDS0165_210310_RAW_cal__ref_\" ->   <|    \"ζ\" -> 0.033577393126   ,  \"τ1\" -> 0.018946820322   ,  \"τS\" -> 0.035749921348   ,  \"τN\" -> 0.004008447047   ,  \"τC\" -> 0.003122429757   ,  \"κ0\" -> 0.000000002680   ,  \"mm1\" -> 0.000093748549   ,  \"mm2\" -> 0.016142439680   ,  \"mm3\" -> 0.046926412611   ,  \"T\" -> 0.430000000000   ,  \"B\" -> 12.000000000000   ,  \"θ\" -> 0.000000000000   ,  \"Reoff\" -> -1313253.012048184870   ,  \"Imoff\" -> 0.000000000000   ,  \"στ1\" -> 0.017565086331   ,  \"στS\" -> 0.001375721175   ,  \"στN\" -> 0.000000000000    |>   , \n\"IDS0165_210310_RAW_cal__sam_\" ->   <|    \"ζ\" -> 0.031945976845   ,  \"τ1\" -> 0.019000922826   ,  \"τS\" -> 0.045624146388   ,  \"τN\" -> 0.005314716063   ,  \"τC\" -> 0.002488383471   ,  \"κ0\" -> 0.000000002954   ,  \"mm1\" -> 0.000073272643   ,  \"mm2\" -> 0.016306894362   ,  \"mm3\" -> 0.057675293464   ,  \"T\" -> 0.430000000000   ,  \"B\" -> 12.000000000000   ,  \"θ\" -> 0.000000000000   ,  \"Reoff\" -> 0.000000000000   ,  \"Imoff\" -> 0.000000000000   ,  \"στ1\" -> 0.000000000000   ,  \"στS\" -> 0.000000000000   ,  \"στN\" -> 0.000000000000    |>   , \n\"IDS0166_210310_RAW_cal__ref_\" ->   <|    \"ζ\" -> 0.026134408941   ,  \"τ1\" -> 0.018837221506   ,  \"τS\" -> 0.029046436266   ,  \"τN\" -> 0.002475934064   ,  \"τC\" -> 0.003637611641   ,  \"κ0\" -> 0.000000003369   ,  \"mm1\" -> 0.000082770074   ,  \"mm2\" -> 0.016386102123   ,  \"mm3\" -> 0.038352149797   ,  \"T\" -> 0.520000000000   ,  \"B\" -> 12.000000000000   ,  \"θ\" -> 0.000000000000   ,  \"Reoff\" -> -406626.506024092435   ,  \"Imoff\" -> 0.000000000000   ,  \"στ1\" -> 0.034768871814   ,  \"στS\" -> 0.001627850434   ,  \"στN\" -> 0.000000000000    |>   , \n\"IDS0166_210310_RAW_cal__sam_\" ->   <|    \"ζ\" -> 0.023031239946   ,  \"τ1\" -> 0.018268814012   ,  \"τS\" -> 0.037269400776   ,  \"τN\" -> 0.002696792890   ,  \"τC\" -> 0.003257395394   ,  \"κ0\" -> 0.000000003720   ,  \"mm1\" -> 0.000067670174   ,  \"mm2\" -> 0.016445281937   ,  \"mm3\" -> 0.045899921957   ,  \"T\" -> 0.520000000000   ,  \"B\" -> 12.000000000000   ,  \"θ\" -> 0.000000000000   ,  \"Reoff\" -> 0.000000000000   ,  \"Imoff\" -> 0.000000000000   ,  \"στ1\" -> 0.000000000000   ,  \"στS\" -> 0.000000000000   ,  \"στN\" -> 0.000000000000    |>   , \n\"IDS0167_210310_RAW_cal__ref_\" ->   <|    \"ζ\" -> 0.026557278794   ,  \"τ1\" -> 0.016933945977   ,  \"τS\" -> 0.022881111855   ,  \"τN\" -> 0.001392473895   ,  \"τC\" -> 0.004119437148   ,  \"κ0\" -> 0.000000003981   ,  \"mm1\" -> 0.000090964667   ,  \"mm2\" -> 0.015177563241   ,  \"mm3\" -> 0.030703081351   ,  \"T\" -> 0.620000000000   ,  \"B\" -> 12.000000000000   ,  \"θ\" -> 0.000000000000   ,  \"Reoff\" -> 0.000000000000   ,  \"Imoff\" -> 0.000000000000   ,  \"στ1\" -> 0.000000000000   ,  \"στS\" -> 0.000000000000   ,  \"στN\" -> 0.000000000000    |>   , \n\"IDS0167_210310_RAW_cal__sam_\" ->   <|    \"ζ\" -> 0.019920170845   ,  \"τ1\" -> 0.016368892412   ,  \"τS\" -> 0.030579536580   ,  \"τN\" -> 0.001736017565   ,  \"τC\" -> 0.004971418152   ,  \"κ0\" -> 0.000000004410   ,  \"mm1\" -> 0.000083939556   ,  \"mm2\" -> 0.015095997595   ,  \"mm3\" -> 0.039119658918   ,  \"T\" -> 0.620000000000   ,  \"B\" -> 12.000000000000   ,  \"θ\" -> 0.000000000000   ,  \"Reoff\" -> 0.000000000000   ,  \"Imoff\" -> 0.000000000000   ,  \"στ1\" -> 0.000000000000   ,  \"στS\" -> 0.000000000000   ,  \"στN\" -> 0.000000000000    |>   , \n\"IDS0168_210310_RAW_cal__ref_\" ->   <|    \"ζ\" -> 0.022041296958   ,  \"τ1\" -> 0.014045615335   ,  \"τS\" -> 0.018889590451   ,  \"τN\" -> 0.000813465770   ,  \"τC\" -> 0.004122617309   ,  \"κ0\" -> 0.000000005540   ,  \"mm1\" -> 0.000073491061   ,  \"mm2\" -> 0.013002629707   ,  \"mm3\" -> 0.025229449010   ,  \"T\" -> 0.810000000000   ,  \"B\" -> 12.000000000000   ,  \"θ\" -> 0.000000000000   ,  \"Reoff\" -> 0.000000000000   ,  \"Imoff\" -> 0.000000000000   ,  \"στ1\" -> 0.000000000000   ,  \"στS\" -> 0.000000000000   ,  \"στN\" -> 0.000000000000    |>   , \n\"IDS0168_210310_RAW_cal__sam_\" ->   <|    \"ζ\" -> 0.017558473054   ,  \"τ1\" -> 0.014545104284   ,  \"τS\" -> 0.022979681288   ,  \"τN\" -> 0.000840829385   ,  \"τC\" -> 0.005228030240   ,  \"κ0\" -> 0.000000006068   ,  \"mm1\" -> 0.000073916527   ,  \"mm2\" -> 0.013750428362   ,  \"mm3\" -> 0.030187552103   ,  \"T\" -> 0.810000000000   ,  \"B\" -> 12.000000000000   ,  \"θ\" -> 0.000000000000   ,  \"Reoff\" -> 0.000000000000   ,  \"Imoff\" -> 0.000000000000   ,  \"στ1\" -> 0.000000000000   ,  \"στS\" -> 0.000000000000   ,  \"στN\" -> 0.000000000000    |>   , \n\"IDS0169_210310_RAW_cal__ref_\" ->   <|    \"ζ\" -> 0.021090283514   ,  \"τ1\" -> 0.013945744068   ,  \"τS\" -> 0.014386606899   ,  \"τN\" -> 0.000345175874   ,  \"τC\" -> 0.004902956629   ,  \"κ0\" -> 0.000000007742   ,  \"mm1\" -> 0.000076221408   ,  \"mm2\" -> 0.013209066715   ,  \"mm3\" -> 0.020605892822   ,  \"T\" -> 1.120000000000   ,  \"B\" -> 12.000000000000   ,  \"θ\" -> 0.000000000000   ,  \"Reoff\" -> 0.000000000000   ,  \"Imoff\" -> 0.000000000000   ,  \"στ1\" -> 0.000000000000   ,  \"στS\" -> 0.000000000000   ,  \"στN\" -> 0.000000000000    |>   , \n\"IDS0169_210310_RAW_cal__sam_\" ->   <|    \"ζ\" -> 0.011916480594   ,  \"τ1\" -> 0.012551282481   ,  \"τS\" -> 0.018233218660   ,  \"τN\" -> 0.000345702746   ,  \"τC\" -> 0.004699451527   ,  \"κ0\" -> 0.000000008451   ,  \"mm1\" -> 0.000044190864   ,  \"mm2\" -> 0.012162820727   ,  \"mm3\" -> 0.023844039179   ,  \"T\" -> 1.120000000000   ,  \"B\" -> 12.000000000000   ,  \"θ\" -> 0.000000000000   ,  \"Reoff\" -> 0.000000000000   ,  \"Imoff\" -> 0.000000000000   ,  \"στ1\" -> 0.000000000000   ,  \"στS\" -> 0.000000000000   ,  \"στN\" -> 0.000000000000    |>   , \n\"IDS0170_210310_RAW_cal__ref_\" ->   <|    \"ζ\" -> 0.021449250230   ,  \"τ1\" -> 0.014564522147   ,  \"τS\" -> 0.008878867204   ,  \"τN\" -> 0.000064984242   ,  \"τC\" -> 0.006207353748   ,  \"κ0\" -> 0.000000012530   ,  \"mm1\" -> 0.000077778127   ,  \"mm2\" -> 0.013872772336   ,  \"mm3\" -> 0.015957015786   ,  \"T\" -> 1.800000000000   ,  \"B\" -> 12.000000000000   ,  \"θ\" -> 0.000000000000   ,  \"Reoff\" -> 0.000000000000   ,  \"Imoff\" -> 0.000000000000   ,  \"στ1\" -> 0.000000000000   ,  \"στS\" -> 0.000000000000   ,  \"στN\" -> 0.000000000000    |>   , \n\"IDS0170_210310_RAW_cal__sam_\" ->   <|    \"ζ\" -> 0.012831327568   ,  \"τ1\" -> 0.013315909415   ,  \"τS\" -> 0.012590836847   ,  \"τN\" -> 0.000065003013   ,  \"τC\" -> 0.005276356243   ,  \"κ0\" -> 0.000000013610   ,  \"mm1\" -> 0.000047406274   ,  \"mm2\" -> 0.013137605540   ,  \"mm3\" -> 0.018225484932   ,  \"T\" -> 1.800000000000   ,  \"B\" -> 12.000000000000   ,  \"θ\" -> 0.000000000000   ,  \"Reoff\" -> 0.000000000000   ,  \"Imoff\" -> 0.000000000000   ,  \"στ1\" -> 0.000000000000   ,  \"στS\" -> 0.000000000000   ,  \"στN\" -> 0.000000000000    |>   , \n\"IDS0171_210310_RAW_cal__ref_\" ->   <|    \"ζ\" -> 0.024633693577   ,  \"τ1\" -> 0.014940694735   ,  \"τS\" -> 0.006137734482   ,  \"τN\" -> 0.000014567254   ,  \"τC\" -> 0.005080683927   ,  \"κ0\" -> 0.000000022488   ,  \"mm1\" -> 0.000067969819   ,  \"mm2\" -> 0.011256263587   ,  \"mm3\" -> 0.015001000908   ,  \"T\" -> 3.100000000000   ,  \"B\" -> 12.000000000000   ,  \"θ\" -> 0.000000000000   ,  \"Reoff\" -> 0.000000000000   ,  \"Imoff\" -> 0.000000000000   ,  \"στ1\" -> 0.000000000000   ,  \"στS\" -> 0.000000000000   ,  \"στN\" -> 0.000000000000    |>   , \n\"IDS0171_210310_RAW_cal__sam_\" ->   <|    \"ζ\" -> 0.019774146838   ,  \"τ1\" -> 0.013257273421   ,  \"τS\" -> 0.007064131508   ,  \"τN\" -> 0.000028000819   ,  \"τC\" -> 0.006942241845   ,  \"κ0\" -> 0.000000023477   ,  \"mm1\" -> 0.000068886863   ,  \"mm2\" -> 0.012935419574   ,  \"mm3\" -> 0.014427582022   ,  \"T\" -> 3.100000000000   ,  \"B\" -> 12.000000000000   ,  \"θ\" -> 0.000000000000   ,  \"Reoff\" -> 0.000000000000   ,  \"Imoff\" -> 0.000000000000   ,  \"στ1\" -> 0.000000000000   ,  \"στS\" -> 0.000000000000   ,  \"στN\" -> 0.000000000000    |>   , \n\"IDS0172_210310_RAW_cal__ref_\" ->   <|    \"ζ\" -> 0.027835388666   ,  \"τ1\" -> 0.013976390421   ,  \"τS\" -> 0.003539188638   ,  \"τN\" -> 0.000003774856   ,  \"τC\" -> 0.004420299329   ,  \"κ0\" -> 0.000000055482   ,  \"mm1\" -> 0.000054408485   ,  \"mm2\" -> 0.007998445403   ,  \"mm3\" -> 0.013985419121   ,  \"T\" -> 5.500000000000   ,  \"B\" -> 12.000000000000   ,  \"θ\" -> 0.000000000000   ,  \"Reoff\" -> 0.000000000000   ,  \"Imoff\" -> 0.000000000000   ,  \"στ1\" -> 0.000000000000   ,  \"στS\" -> 0.000000000000   ,  \"στN\" -> 0.000000000000    |>   , \n\"IDS0172_210310_RAW_cal__sam_\" ->   <|    \"ζ\" -> 0.029251354442   ,  \"τ1\" -> 0.014634751206   ,  \"τS\" -> 0.003873958746   ,  \"τN\" -> 0.000007000487   ,  \"τC\" -> 0.006827504775   ,  \"κ0\" -> 0.000000056438   ,  \"mm1\" -> 0.000072018576   ,  \"mm2\" -> 0.010723236476   ,  \"mm3\" -> 0.014661483476   ,  \"T\" -> 5.500000000000   ,  \"B\" -> 12.000000000000   ,  \"θ\" -> 0.000000000000   ,  \"Reoff\" -> 0.000000000000   ,  \"Imoff\" -> 0.000000000000   ,  \"στ1\" -> 0.000000000000   ,  \"στS\" -> 0.000000000000   ,  \"στN\" -> 0.000000000000    |>   , \n\"IDS0181_210310_RAW_cal__ref_\" ->   <|    \"ζ\" -> 0.207215393706   ,  \"τ1\" -> 0.071614759547   ,  \"τS\" -> 0.033372244593   ,  \"τN\" -> 0.118024087364   ,  \"τC\" -> 0.000911312721   ,  \"κ0\" -> 0.000000000896   ,  \"mm1\" -> 0.000153514785   ,  \"mm2\" -> 0.012095986783   ,  \"mm3\" -> 0.243044553189   ,  \"T\" -> 0.179000000000   ,  \"B\" -> 12.000000000000   ,  \"θ\" -> 90.000000000000   ,  \"Reoff\" -> -48057142.857142858200   ,  \"Imoff\" -> 0.000000000000   ,  \"στ1\" -> 0.006739310005   ,  \"στS\" -> 0.001034889323   ,  \"στN\" -> 0.008466753702    |>   , \n\"IDS0181_210310_RAW_cal__sam_\" ->   <|    \"ζ\" -> 0.161975781729   ,  \"τ1\" -> 0.073089805113   ,  \"τS\" -> 0.045018408115   ,  \"τN\" -> 0.161987434028   ,  \"τC\" -> 0.001482104484   ,  \"κ0\" -> 0.000000001038   ,  \"mm1\" -> 0.000201615809   ,  \"mm2\" -> 0.012976126678   ,  \"mm3\" -> 0.301929942357   ,  \"T\" -> 0.179000000000   ,  \"B\" -> 12.000000000000   ,  \"θ\" -> 90.000000000000   ,  \"Reoff\" -> 0.000000000000   ,  \"Imoff\" -> 0.000000000000   ,  \"στ1\" -> 0.000000000000   ,  \"στS\" -> 0.000000000000   ,  \"στN\" -> 0.000000000000    |>   , \n\"IDS0183_210310_RAW_cal__ref_\" ->   <|    \"ζ\" -> 0.385034678863   ,  \"τ1\" -> 0.098452305085   ,  \"τS\" -> 0.050647974835   ,  \"τN\" -> 0.644878234475   ,  \"τC\" -> 0.000955383413   ,  \"κ0\" -> 0.000000000435   ,  \"mm1\" -> 0.000262906289   ,  \"mm2\" -> 0.006607789278   ,  \"mm3\" -> 1.055864912884   ,  \"T\" -> 0.120000000000   ,  \"B\" -> 12.000000000000   ,  \"θ\" -> 90.000000000000   ,  \"Reoff\" -> -152673469.387755096000   ,  \"Imoff\" -> 0.000000000000   ,  \"στ1\" -> 0.036947349367   ,  \"στS\" -> 0.009183803549   ,  \"στN\" -> 0.178905609982    |>   , \n\"IDS0183_210310_RAW_cal__sam_\" ->   <|    \"ζ\" -> 0.300863384227   ,  \"τ1\" -> 0.104924004009   ,  \"τS\" -> 0.071070599729   ,  \"τN\" -> 0.992887187112   ,  \"τC\" -> 0.001721587800   ,  \"κ0\" -> 0.000000000548   ,  \"mm1\" -> 0.000392216822   ,  \"mm2\" -> 0.006637384427   ,  \"mm3\" -> 1.483679717825   ,  \"T\" -> 0.120000000000   ,  \"B\" -> 12.000000000000   ,  \"θ\" -> 90.000000000000   ,  \"Reoff\" -> 0.000000000000   ,  \"Imoff\" -> 0.000000000000   ,  \"στ1\" -> 0.000000000000   ,  \"στS\" -> 0.000000000000   ,  \"στN\" -> 0.000000000000    |>   , \n\"IDS0184_210310_RAW_cal__ref_\" ->   <|    \"ζ\" -> 0.275825823442   ,  \"τ1\" -> 0.091430628427   ,  \"τS\" -> 0.045538598654   ,  \"τN\" -> 0.259515671853   ,  \"τC\" -> 0.000892837832   ,  \"κ0\" -> 0.000000000649   ,  \"mm1\" -> 0.000190693778   ,  \"mm2\" -> 0.011443271469   ,  \"mm3\" -> 0.469885616877   ,  \"T\" -> 0.148000000000   ,  \"B\" -> 12.000000000000   ,  \"θ\" -> 90.000000000000   ,  \"Reoff\" -> -79934693.877551019200   ,  \"Imoff\" -> 0.000000000000   ,  \"στ1\" -> 0.016644868561   ,  
